vi "SV TDMS Write.vi"   [LabVIEW 2017]
doc: "Writes data to the specified .tdms file in a format specific to the polymorphic instance. Wire data to the <B>scaled signal [EU]</B> input to determine the polymorphic instance to use or manually select the instance."
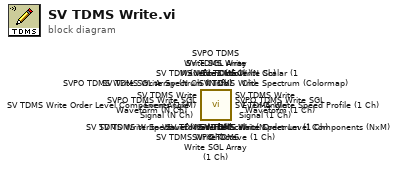
[diagram p0: block diagram]
diagram:
  n1 = call <vilib>:"SV TDMS Write Scalar (N Ch).vi"() -> ()  [unwired: 12 in, 4 out]
  n2 = call <vilib>:"SV TDMS Write Scalar (1 Ch).vi"() -> ()  [unwired: 12 in, 4 out]
  n3 = call <vilib>:"SVPO TDMS Write SGL Waveform (N Ch).vi"() -> ()  [unwired: 13 in, 3 out]
  n4 = call <vilib>:"SVPO TDMS Write SGL Waveform (1 Ch).vi"() -> ()  [unwired: 13 in, 3 out]
  n5 = call <vilib>:"SVPO TDMS Write SGL Array (N Ch N Info).vi"() -> ()  [unwired: 13 in, 3 out]
  n6 = call <vilib>:"SVPO TDMS Write SGL Array (N Ch 1 Info).vi"() -> ()  [unwired: 13 in, 3 out]
  n7 = call <vilib>:"SVPO TDMS Write SGL Array (1 Ch).vi"() -> ()  [unwired: 13 in, 3 out]
  n8 = call <vilib>:"SV TDMS Write Order Level Components (NxM).vi"() -> ()  [unwired: 12 in, 4 out]
  n9 = call <vilib>:"SV TDMS Write Order Level Components (1xM).vi"() -> ()  [unwired: 12 in, 4 out]
  n10 = call <vilib>:"SV TDMS Write Speed Profile (1 Ch).vi"() -> ()  [unwired: 12 in, 4 out]
  n11 = call <vilib>:"SV TDMS Write Spectrum (Waterfall).vi"() -> ()  [unwired: 12 in, 4 out]
  n12 = call <vilib>:"SV TDMS Write Spectrum (Colormap).vi"() -> ()  [unwired: 13 in, 3 out]
  n13 = call <vilib>:"SV TDMS Write Octave (N Ch).vi"() -> ()  [unwired: 12 in, 4 out]
  n14 = call <vilib>:"SV TDMS Write Octave (1 Ch).vi"() -> ()  [unwired: 12 in, 4 out]
  n15 = call <vilib>:"SV TDMS Write Even-Angle Signal (N Ch).vi"() -> ()  [unwired: 12 in, 4 out]
  n16 = call <vilib>:"SV TDMS Write Even-Angle Signal (1 Ch).vi"() -> ()  [unwired: 12 in, 4 out]
  n17 = call <vilib>:"SV TDMS Write Spectrum (N Ch).vi"() -> ()  [unwired: 12 in, 4 out]
  n18 = call <vilib>:"SV TDMS Write Spectrum (1 Ch).vi"() -> ()  [unwired: 12 in, 4 out]
  n19 = call <vilib>:"SV TDMS Write Waveform (N Ch).vi"() -> ()  [unwired: 12 in, 4 out]
  n20 = call <vilib>:"SV TDMS Write Waveform (1 Ch).vi"() -> ()  [unwired: 12 in, 4 out]
